vi "Initialize-intruments.vi"(0 "Initialize":bool, 1 "Status":T1={"CCD - Symphony Status 2"={"CCD - Status"="", "Error"=FALSE, "Initialized"=FALSE}, "Common: CCD 2"={"ID: CCD"=refnum, "Name"="ccd de test", "FirmwareVersion"="V1.89  CCD_3000", "activeXPixels"=1024, "activeYPixels"=256, "ADC Number"=[0], "ADC description"=[""], "Gain Number"=[0], "Gain description"=[""]}, "Monochromator - HR460 Status 2"={"Spectral Position"=0.0, "Spectral Unit"="", "Groove Density"=0.0, "Slit Width"=0.0, "Slit Unit"="", "Error"=FALSE, "Initialized"=FALSE}, "Stage - PI C844 Status 2"={" Identification Message "="", "Error"=FALSE, "Initialized"=FALSE}, "Temperature Controller - Status 2"={"Initialized"=FALSE, "Sample Temperature"=0.0, "Heater"=0, "Set Point"=20.0, "Error"=FALSE, "Sample Channel"=0, "Sample Channel Units"=0, "Unit"="Kelvin"}} {"Temperature Controller - Status 2"."Sample Channel Units" items=["Kelvin", "Celsius", "Sensor Units"]; "Temperature Controller - Status 2"."Sample Channel" items=["Sensor A", "Sensor B"]; "Temperature Controller - Status 2"."Heater" scale=0.0..100.0}, 5 "Instruments":T4, 7 "Monochromator - HR460 Control":T3, 9 "Stage - PI C844 Control":T6={" RS-232 Port Select "=0, " Interface Select "=1, "  P-term         I-term         D-term         Accel."=[[275, 120, 100, 2000000], [250, 40, 800, 2000000]]} {"Interface Select" items=["IEEE488", "RS-232"]; "RS-232 Port Select" items=["COM1", "COM2", "COM3", "COM4"]}, 11 "Temperature Controller - Control":T5={"VISA Resource Name"="GPIB0::12::INSTR", "Control Channel"=0, "Sample Channel Units"=0} {"Sample Channel Units" items=["Kelvin", "Celsius", "Sensor Units"]; "Control Channel" items=["Sensor A", "Sensor B"]}, 12 "error in (no error)":errorcluster) -> (3 "Common: CCD":T10={"ID: CCD"=refnum, "Name"="ccd de test", "FirmwareVersion"="V1.89  CCD_3000", "activeXPixels"=1024, "activeYPixels"=256, "ADC Number"=[], "ADC description"=[], "Gain Number"=[], "Gain description"=[]}, 4 "CCD - Symphony Status":T2, 6 "Shutter?":bool, 8 "Monochromator - HR460 Status":T9, 10 "Stage - PI C844 Status":T8, 14 "error out":errorcluster, 15 "Temperature Controller - Status":T7={"Initialized"=FALSE, "Sample Temperature"=0.0, "Heater"=0, "Set Point"=20.0, "Error"=FALSE, "Sample Channel"=0, "Sample Channel Units"=0, "Unit"="Kelvin"} {"Sample Channel Units" items=["Kelvin", "Celsius", "Sensor Units"]; "Sample Channel" items=["Sensor A", "Sensor B"]; "Heater" scale=0.0..100.0})   [LabVIEW 2009]
uses:
  lvmonos_LV7.1_all GPIB and RS232/Isa_user.llb/Spectrometer Status.GBL
  lvmonos_LV7.1_all GPIB and RS232/Isa_user.llb/SPECTROMETER SETUP.GBL
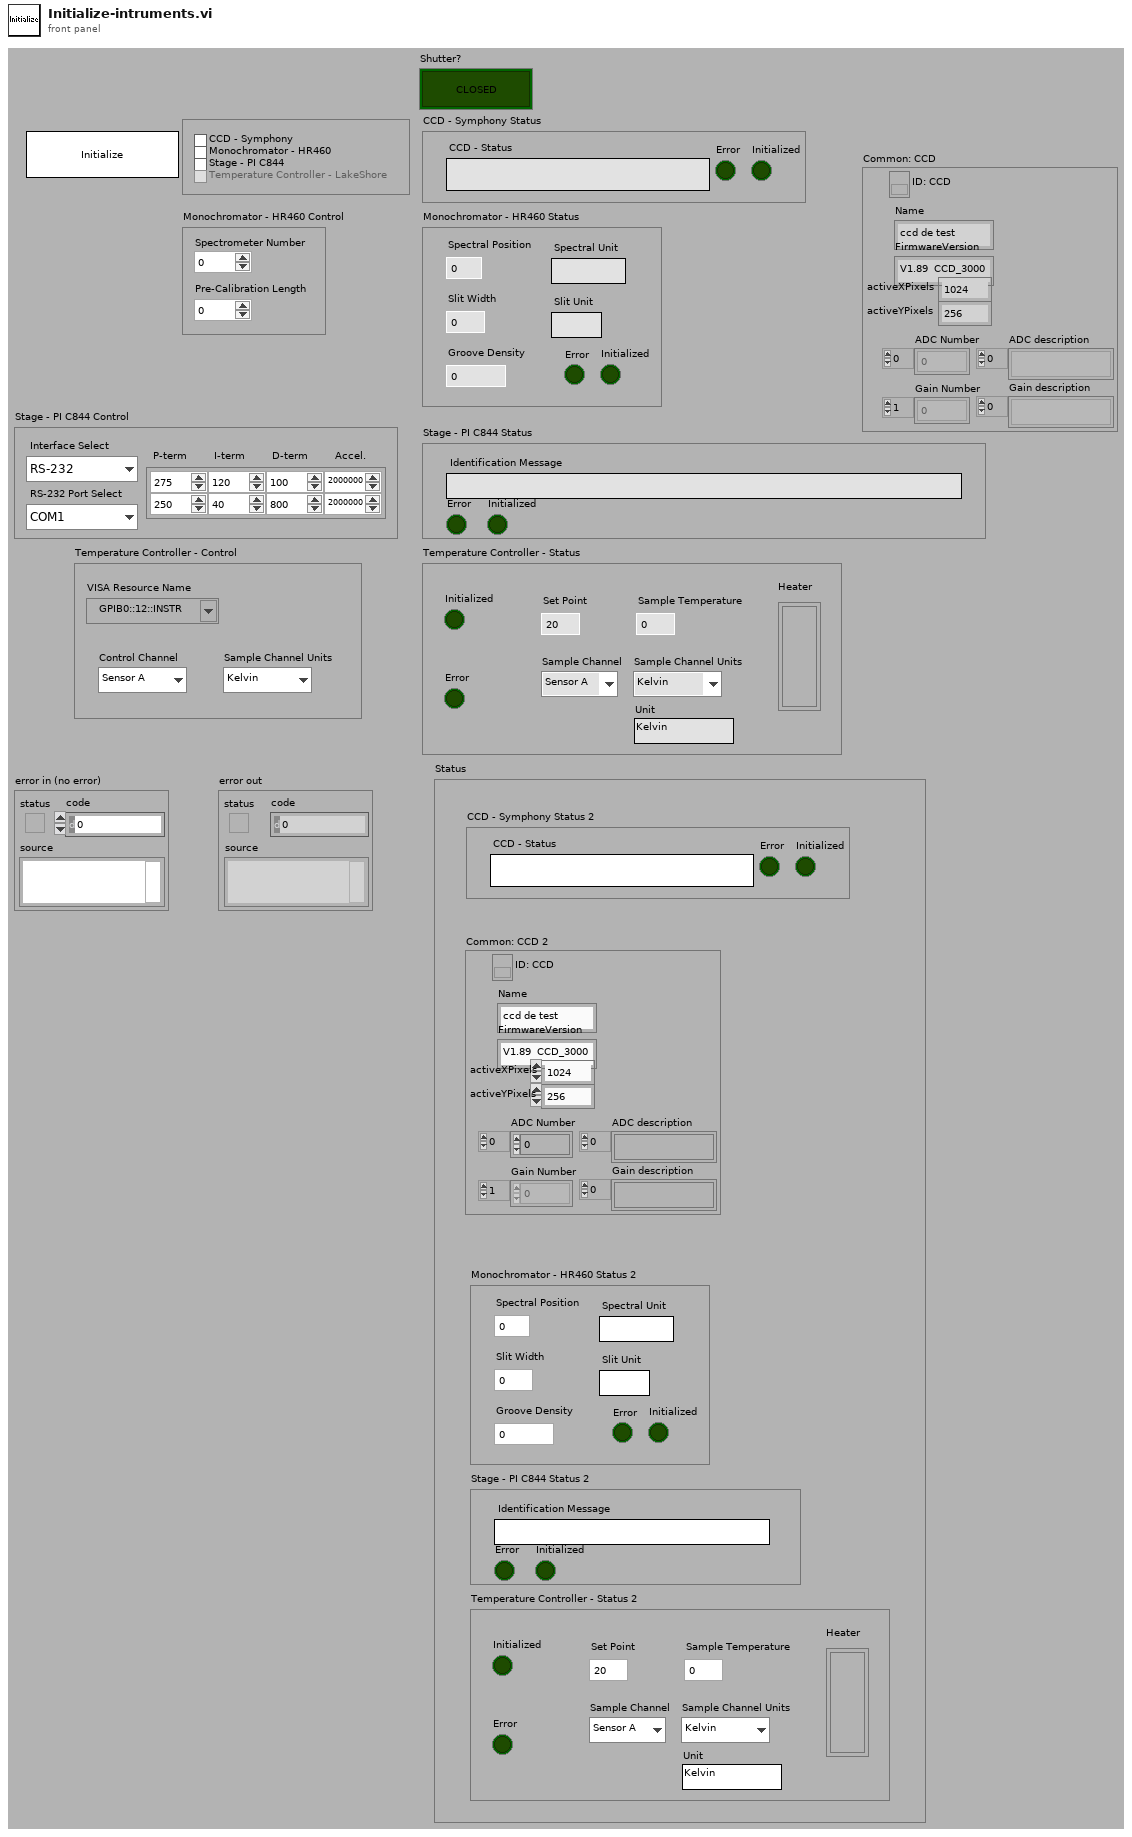
[diagram p1: front panel]
types:
  T1 = cluster{"CCD - Symphony Status 2":cluster{"CCD - Status":string, "Error":bool, "Initialized":bool}, "Common: CCD 2":cluster{"ID: CCD":refnum<k7>, "Name":string, "FirmwareVersion":string, "activeXPixels":i32, "activeYPixels":i32, "ADC Number":i32[], "ADC description":string[], "Gain Number":i32[], "Gain description":string[]}, "Monochromator - HR460 Status 2":cluster{"Spectral Position":dbl, "Spectral Unit":string, "Groove Density":dbl, "Slit Width":dbl, "Slit Unit":string, "Error":bool, "Initialized":bool}, "Stage - PI C844 Status 2":cluster{" Identification Message ":string, "Error":bool, "Initialized":bool}, "Temperature Controller - Status 2":cluster{"Initialized":bool, "Sample Temperature":dbl, "Heater":u8, "Set Point":dbl, "Error":bool, "Sample Channel":u16, "Sample Channel Units":u16, "Unit":string}}
  T2 = cluster{"CCD - Status":string, "Error":bool, "Initialized":bool}
  T3 = cluster{"Spectrometer Number":i32, "Pre-Calibration Length":dbl}
  T4 = cluster{"CCD - Symphony":bool, "Monochromator - HR460":bool, "Stage - PI C844":bool, "Temperature Controller - LakeShore":bool}
  T5 = cluster{"VISA Resource Name":refnum<visa-resource-name>, "Control Channel":u16, "Sample Channel Units":u16}
  T6 = cluster{" RS-232 Port Select ":i32, " Interface Select ":u8, "  P-term         I-term         D-term         Accel.":u32[][]}
  T7 = cluster{"Initialized":bool, "Sample Temperature":dbl, "Heater":u8, "Set Point":dbl, "Error":bool, "Sample Channel":u16, "Sample Channel Units":u16, "Unit":string}
  T8 = cluster{" Identification Message ":string, "Error":bool, "Initialized":bool}
  T9 = cluster{"Spectral Position":dbl, "Spectral Unit":string, "Groove Density":dbl, "Slit Width":dbl, "Slit Unit":string, "Error":bool, "Initialized":bool}
  T10 = cluster{"ID: CCD":refnum<k7>, "Name":string, "FirmwareVersion":string, "activeXPixels":i32, "activeYPixels":i32, "ADC Number":i32[], "ADC description":string[], "Gain Number":i32[], "Gain description":string[]}
  T11 = cluster{"Spectrometer Number":enum32{"Index Zero", "Index One"}, "Communication Parameters":cluster{"Comm Interface":u16, "GPIB Bus":i16, "GPIB Address":i16, "Serial Com Port":i32}, "Calibration":bool, "Groove Density":dbl[], "Blaze Wavelength":dbl[], "Base Grating":dbl, "Steps / Spectral Unit":dbl, "Backlash (Spectral Unit)":dbl, "Min Limit (Spectral Unit)":dbl, "Max Limit (Spectral Unit)":dbl, "Spectral Unit":string, "Slit Installation":cluster{"Axial Entrance":bool, "Lateral Entrance":bool, "Axial Exit":bool, "Lateral Exit":bool}, " Steps / Slit Unit":dbl, "Backlash (Slit Unit)":dbl, "Slit  Unit":string, " Max Limit (Slit Unit)":dbl, " Min Limit (Slit Unit)":dbl, "Drive Type":enum32{"Step", "Wavelength "}}[]
  T12 = cluster{"Spectrometer Number":enum32{"Index Zero", "Index One"}, "Communication Parameters":cluster{"Comm Interface":u16, "GPIB Bus":i16, "GPIB Address":i16, "Serial Com Port":i32}, "Calibration":bool, "Groove Density":dbl[], "Blaze Wavelength":dbl[], "Base Grating":dbl, "Steps / Spectral Unit":dbl, "Backlash (Spectral Unit)":dbl, "Min Limit (Spectral Unit)":dbl, "Max Limit (Spectral Unit)":dbl, "Spectral Unit":string, "Slit Installation":cluster{"Axial Entrance":bool, "Lateral Entrance":bool, "Axial Exit":bool, "Lateral Exit":bool}, " Steps / Slit Unit":dbl, "Backlash (Slit Unit)":dbl, "Slit  Unit":string, " Max Limit (Slit Unit)":dbl, " Min Limit (Slit Unit)":dbl, "Drive Type":enum32{"Step", "Wavelength "}}
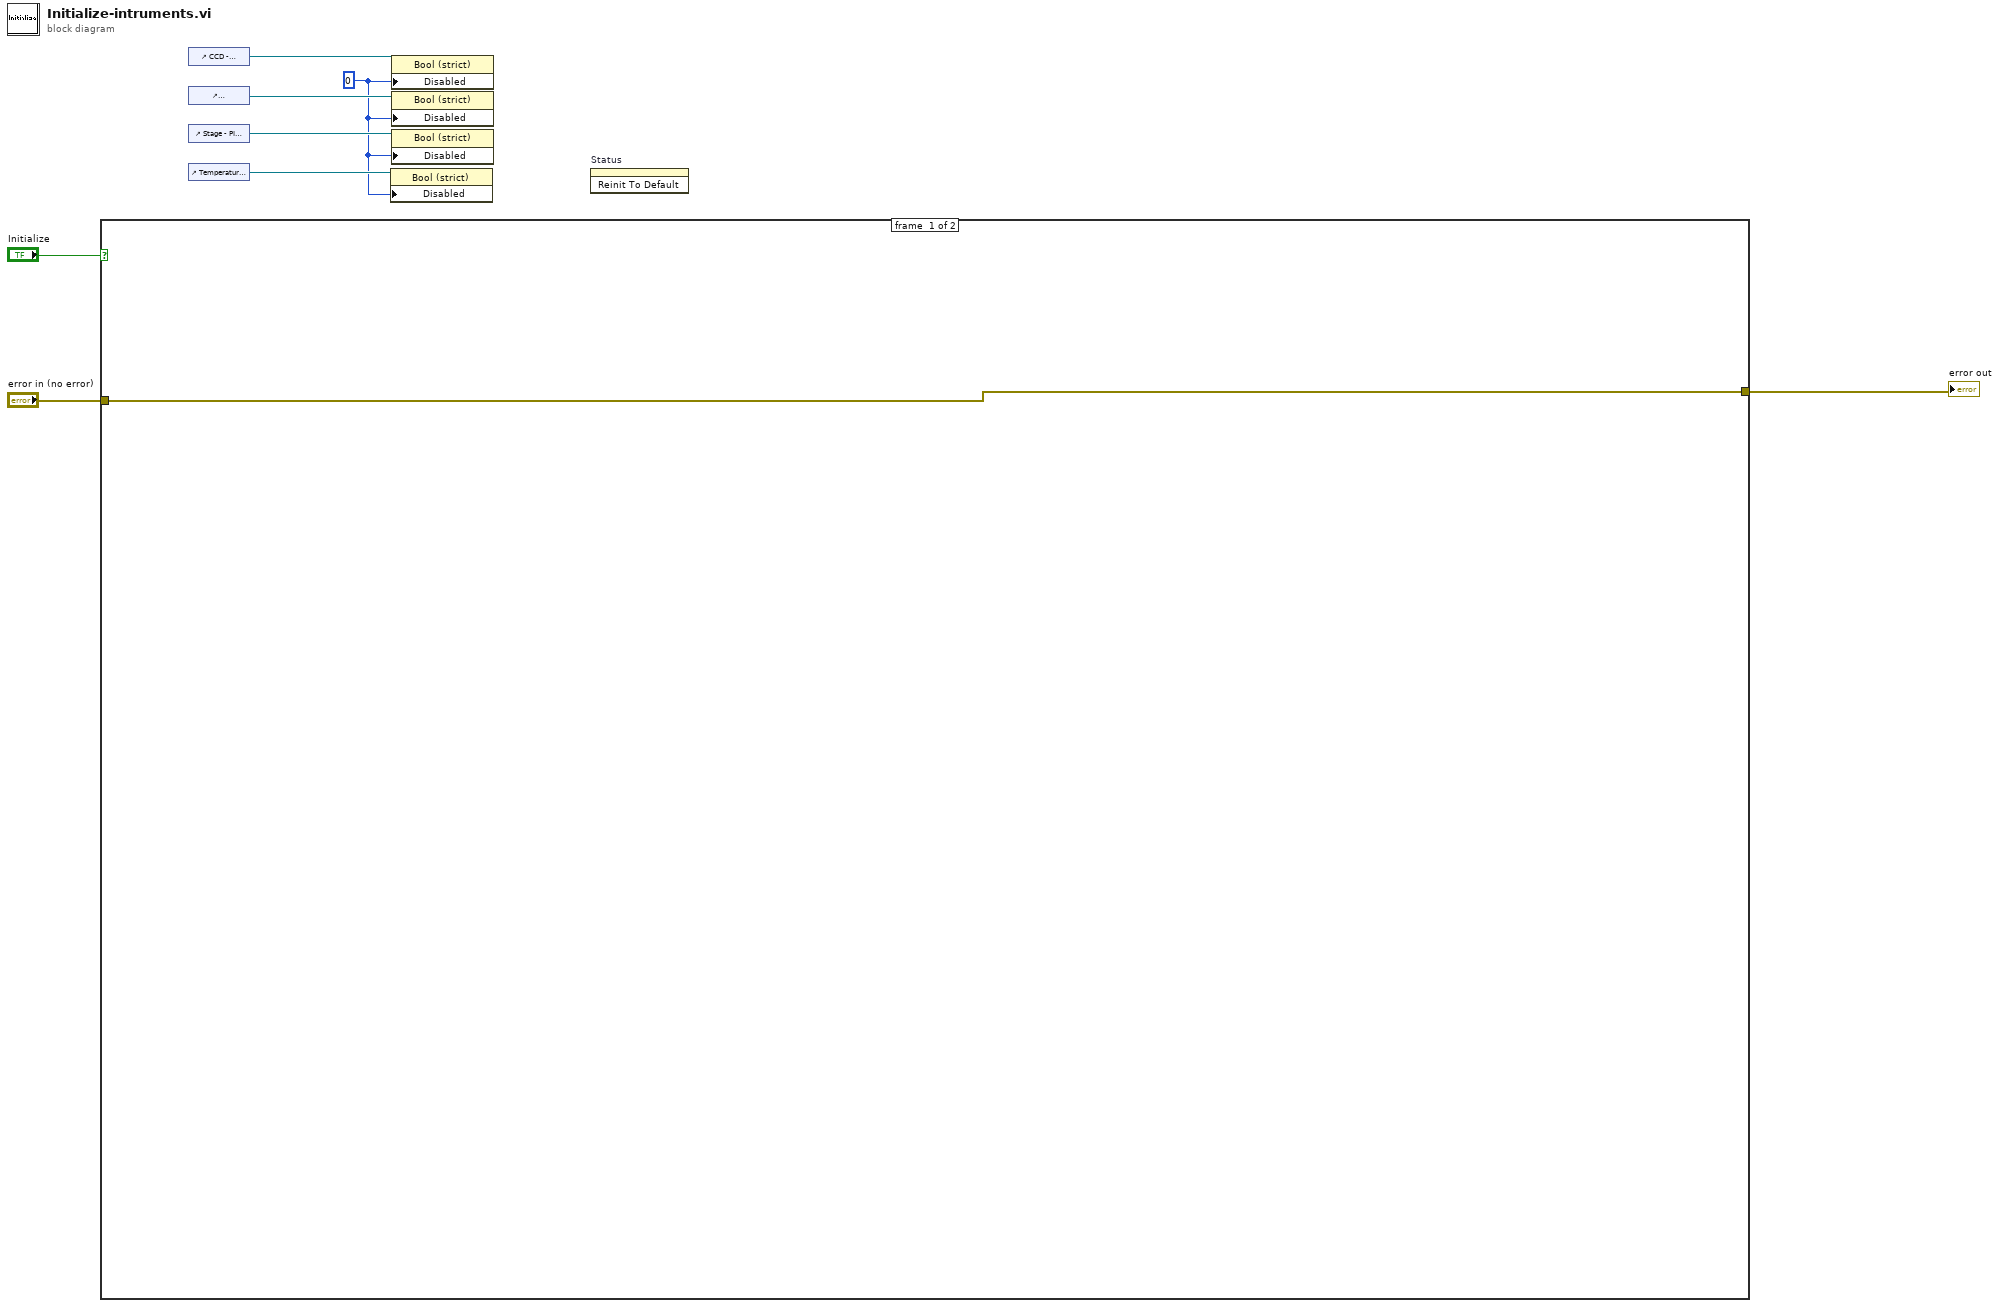
[diagram p0: block diagram]
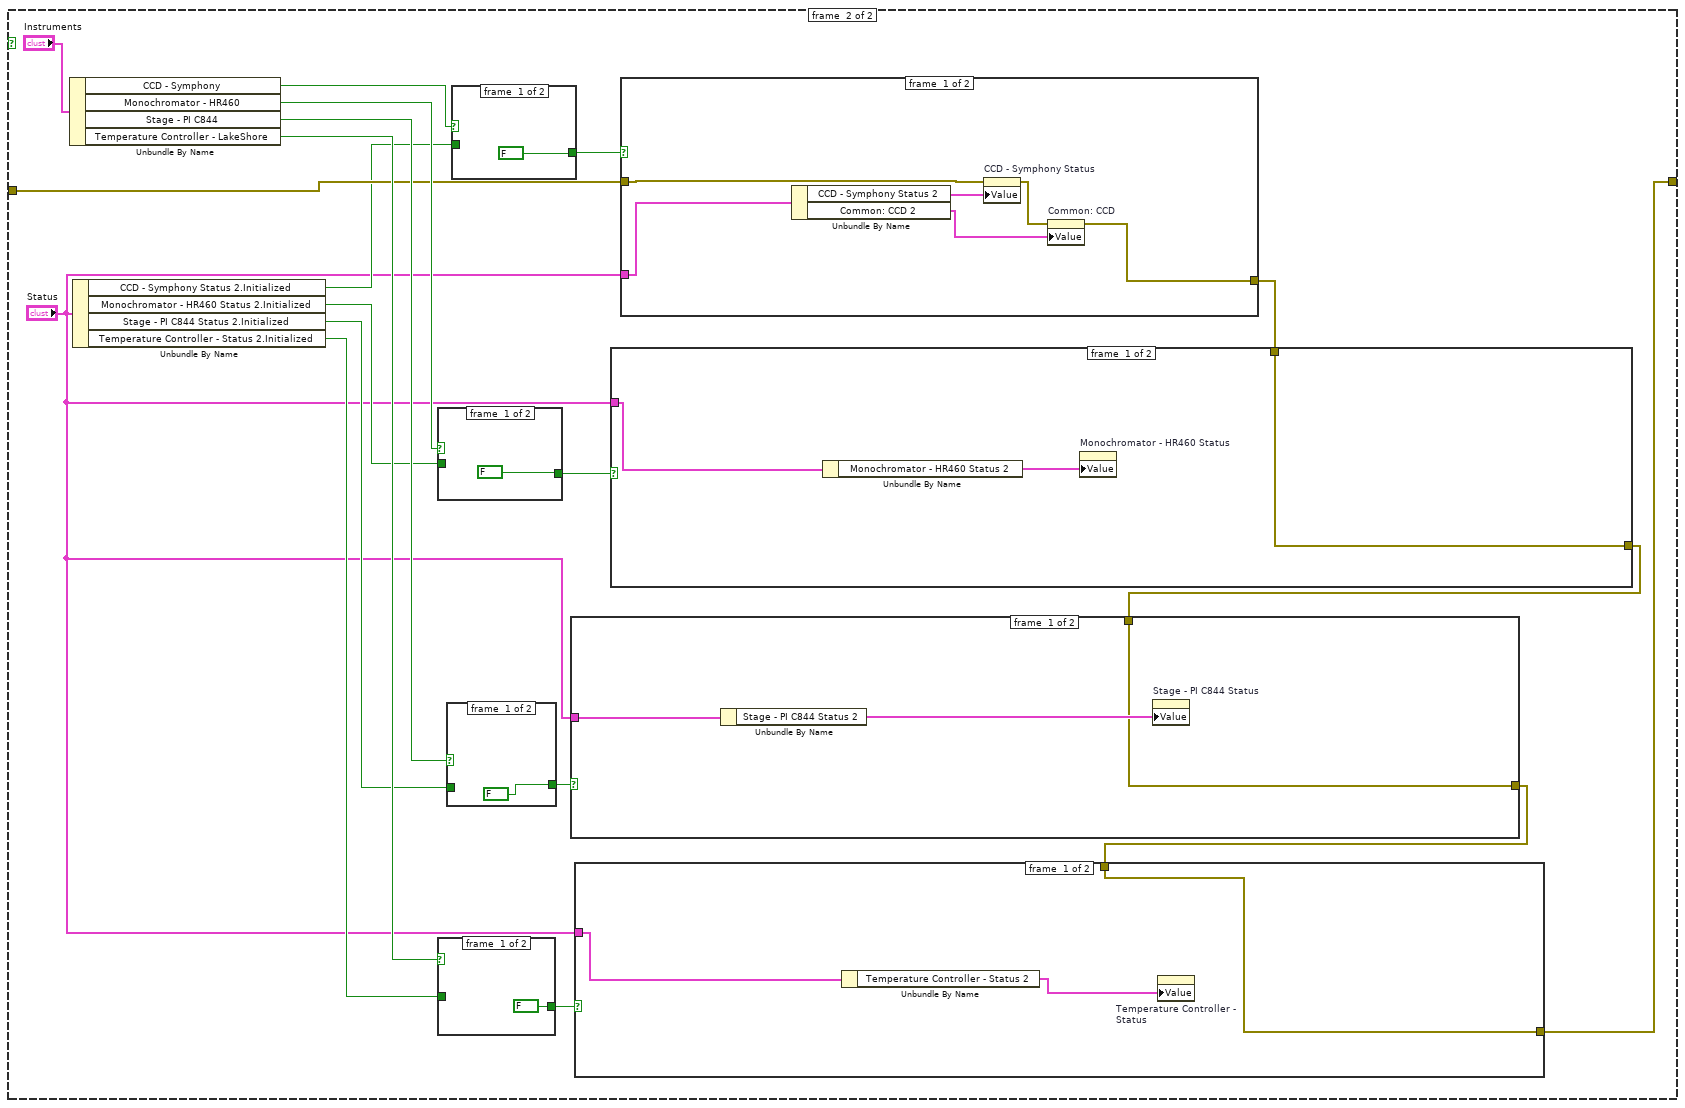
[diagram p2: hidden frame]
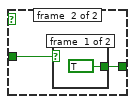
[diagram p3: hidden frame]
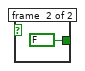
[diagram p4: hidden frame]
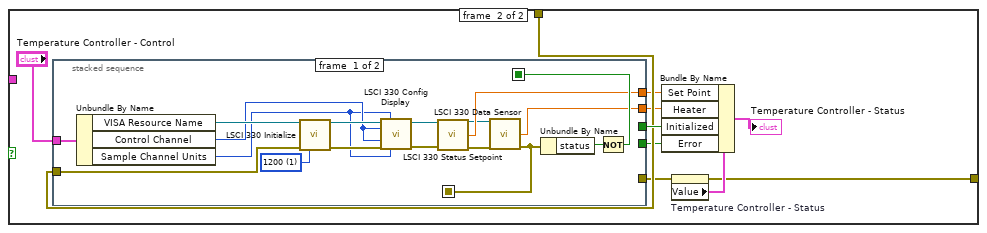
[diagram p5: hidden frame]
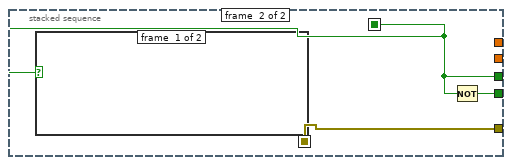
[diagram p6: hidden frame]
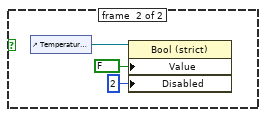
[diagram p7: hidden frame]
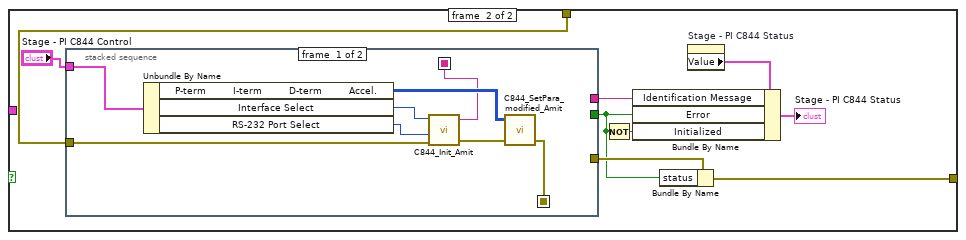
[diagram p8: hidden frame]
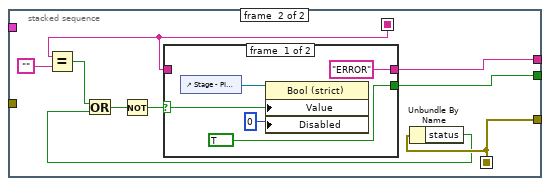
[diagram p9: hidden frame]
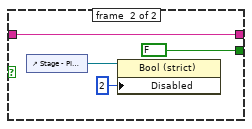
[diagram p10: hidden frame]
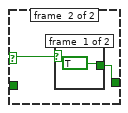
[diagram p11: hidden frame]
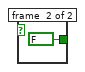
[diagram p12: hidden frame]
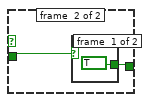
[diagram p13: hidden frame]
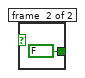
[diagram p14: hidden frame]
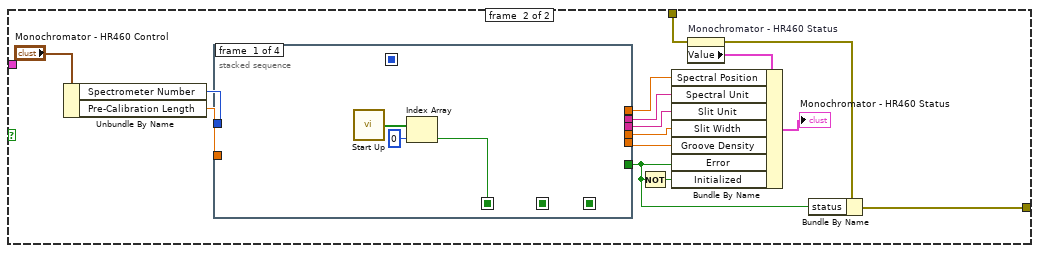
[diagram p15: hidden frame]
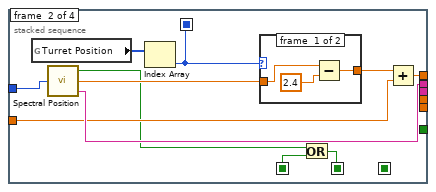
[diagram p16: hidden frame]
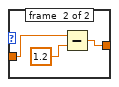
[diagram p17: hidden frame]
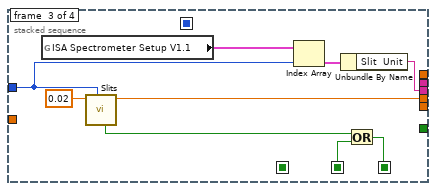
[diagram p18: hidden frame]
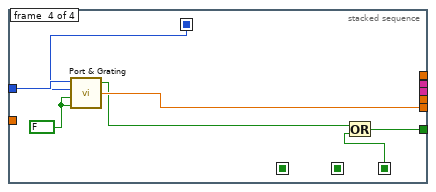
[diagram p19: hidden frame]
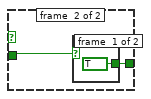
[diagram p20: hidden frame]
diagram:
  w1 = u8 0 ("Disabled")
  n1 = case shown="True" "Initialize" {
    tunnel: [w9 w15] -> w6
    tunnel: "error in (no error)" -> [w9 w23]
    frame #0 {
    }
    frame #1 {
      n2 = Unbundle By Name("Instruments") -> ("CCD - Symphony"=w24:bool, "Monochromator - HR460"=w25:bool, "Stage - PI C844"=w26:bool, "Temperature Controller - LakeShore"=w27:bool)
      n3 = Unbundle By Name("Status") -> ("CCD - Symphony Status 2.Initialized"=w14:bool, "Monochromator - HR460 Status 2.Initialized"=w13:bool, "Stage - PI C844 Status 2.Initialized"=w12:bool, "Temperature Controller - Status 2.Initialized"=w11:bool)
      n4 = case shown="False" w25 {
        tunnel: [FALSE w115] -> w21
        tunnel: w13 -> [_ w114]
        frame #0 {
        }
        frame #1 {
          n5 = case shown="True" w114 {
            tunnel: [TRUE FALSE] -> w115
            frame #0 {
            }
            frame #1 {
            }
          }
        }
      }
      n6 = case shown="False" w27 {
        tunnel: [FALSE w31] -> w19
        tunnel: w11 -> [_ w30]
        frame #0 {
        }
        frame #1 {
          n7 = case shown="True" w30 {
            tunnel: [TRUE FALSE] -> w31
            frame #0 {
            }
            frame #1 {
            }
          }
        }
      }
      n8 = case shown="True" w26 {
        tunnel: [FALSE w110] -> w20
        tunnel: w12 -> [_ w109]
        frame #0 {
        }
        frame #1 {
          n9 = case shown="False" w109 {
            tunnel: [TRUE FALSE] -> w110
            frame #0 {
            }
            frame #1 {
            }
          }
        }
      }
      n10 = case shown="False" w24 {
        tunnel: [FALSE w174] -> w22
        tunnel: w14 -> [_ w173]
        frame #0 {
        }
        frame #1 {
          n11 = case shown="False" w173 {
            tunnel: [TRUE FALSE] -> w174
            frame #0 {
            }
            frame #1 {
            }
          }
        }
      }
      n12 = case shown="True" w22 {
        tunnel: w23 -> [w180 w186]
        tunnel: [w177 w184] -> w18
        tunnel: "Status" -> [w182 _]
        frame #0 {
          n13 = Unbundle By Name(w182) -> ("CCD - Symphony Status 2"=w181:T2, "Common: CCD 2"=w179:T10)
          n14 = property on="CCD - Symphony Status" class="Clust (strict)"(error in=w180, "Value"=w181) -> (error out=w178:errorcluster)  [unwired: 1 in, 1 out]
          n15 = property on="Common: CCD" class="Clust (strict)"(error in=w178, "Value"=w179) -> (error out=w177:errorcluster)  [unwired: 1 in, 1 out]
        }
        frame #1 {
          n16 = stacked-sequence {
            seq-local: [_ w194 _] -> [_ _ w196]
            seq-local: [w187 _ _] -> [_ w191 _]
            tunnel: [_ _ w196] -> w185
            tunnel: w186 -> [w187 _ _]
            tunnel: [_ _ w195] -> w183
            frame #0 {
              w188 = FALSE
              n17 = Bundle("Initializing...", w188, w188) -> (→"CCD - Symphony Status":cluster{string, bool, bool})  [unwired: 1 in]
            }
            frame #1 {
              n18 = call "CCD Initialize-Amit.vi"("error in (no error)"=w191) -> ("error out"=w194:errorcluster, "Shutter?"=→"Shutter?":bool, "Common: CCD"=→"Common: CCD":T10)  [unwired: 7 in, 1 out]
            }
            frame #2 {
              n19 = Unbundle By Name(w196) -> ("status"=w195:bool)
              n20 = case shown="True" w195 {
                tunnel: w195 -> [w198 w204]
                frame #0 {
                  w197 = TRUE ("Value")
                  n21 = control-ref of="CCD - Symphony"() -> (w200:refnum<vi>)
                  n22 = property class="Bool (strict)"(reference=w200, "Disabled"=u8 2, "Value"=w197) -> ()  [unwired: 1 in, 2 out]
                  n23 = Bundle("CCD Initialized!!!  :-)", "status"=w198, "Value"=w197) -> (w202:cluster{string, "status":bool, "Value":bool})  [unwired: 1 in]
                  n24 = property on="CCD - Symphony Status" class="Clust (strict)"("Value"=w202) -> ()  [unwired: 2 in, 2 out]
                }
                frame #1 {
                  w203 = FALSE ("Value")
                  n25 = control-ref of="CCD - Symphony"() -> (w206:refnum<vi>)
                  n26 = property class="Bool (strict)"(reference=w206, "Value"=w203, "Disabled"=u8 0) -> ()  [unwired: 1 in, 2 out]
                  n27 = Bundle("Initialization Failed :-( ", "status"=w204, "Value"=w203) -> (w208:cluster{string, "status":bool, "Value":bool})  [unwired: 1 in]
                  n28 = property on="CCD - Symphony Status" class="Clust (strict)"("Value"=w208) -> ()  [unwired: 2 in, 2 out]
                }
              }
            }
          }
          n29 = Bundle By Name(cluster=w185, "status"=w183) -> (w184:errorcluster)
        }
      }
      n30 = case shown="False" w21 {
        tunnel: [w118 w121] -> w17
        tunnel: w18 -> [w118 w125]
        tunnel: "Status" -> [w120 _]
        frame #0 {
          n31 = Unbundle By Name(w120) -> ("Monochromator - HR460 Status 2"=w119:T9)
          n32 = property on="Monochromator - HR460 Status" class="Clust (strict)"("Value"=w119) -> ()  [unwired: 2 in, 2 out]
        }
        frame #1 {
          n33 = Unbundle By Name("Monochromator - HR460 Control") -> ("Spectrometer Number"=w127:i32, "Pre-Calibration Length"=w126:dbl)
          n34 = stacked-sequence {
            seq-local: [_ w146 _ _] -> [_ _ _ w170]
            seq-local: [w136 _ _ _] -> [_ w141 _ _]
            seq-local: [_ w139 _ _] -> [_ _ w158 _]
            seq-local: [_ _ w156 _] -> [_ _ _ w166]
            tunnel: w127 -> [_ w147 w162 w171]
            tunnel: [_ w144 _ _] -> w135
            tunnel: [_ w143 _ _] -> w134
            tunnel: [_ _ w160 _] -> w133
            tunnel: [_ _ w159 _] -> w132
            tunnel: [_ _ _ w168] -> w131
            tunnel: w126 -> [_ w142 _ _]
            tunnel: [_ _ _ w165] -> w122
            frame #0 {
              n35 = call "Start Up.VI"() -> ("Error List"=w138:bool[])  [unwired: 1 in, 2 out]
              n36 = Index Array(array=w138, index=0) -> (element=w136:bool)
            }
            frame #1 {
              n37 = global read "Spectrometer Status.GBL" "Turret Position"() -> (w149:i32[])
              n38 = call "Spectral Position.VI"("Spectrometer Number"=w147) -> ("Error"=w140:bool, "Present Position"=w148:dbl, "Spectral Unit"=w143:string)
              n39 = Index Array(array=w149) -> (element=w146:i32)  [unwired: 1 in]
              n40 = case shown="1, Default" w146 {
                tunnel: [w152 w154] -> w145
                tunnel: w148 -> [w151 w153]
                frame #0 {
                  n41 = Subtract(x=w151, y=2.4) -> (x-y=w152:dbl)
                }
                frame #1 {
                  n42 = Subtract(x=w153, y=1.2) -> (x-y=w154:dbl)
                }
              }
              n43 = Or(x=w140, y=w141) -> (x .or. y?=w139:bool)
              n44 = Add(x=w145, y=w142) -> (x+y=w144:dbl)
            }
            frame #2 {
              n45 = global read "SPECTROMETER SETUP.GBL" "ISA Spectrometer Setup V1.1"() -> (w163:T11)
              n46 = call "Slits.VI"("Spectrometer Number"=w162, "Axial Entrance"=0.02) -> ("Axial Entrance"=w159:dbl, "Error"=w157:bool)  [unwired: 3 in, 3 out]
              n47 = Index Array(array=w163, index=w162) -> (element=w161:T12)
              n48 = Unbundle By Name(w161) -> ("Slit  Unit"=w160:string)
              n49 = Or(x=w157, y=w158) -> (x .or. y?=w156:bool)
            }
            frame #3 {
              w169 = FALSE
              n50 = call "Port & Grating.VI"("Exit Mirror Pos"=w169, "Entrance Mirror Pos"=w169, "Turret Pos"=w170, "Spectrometer Number"=w171) -> ("Groove Density"=w168:dbl, "Error"=w167:bool)  [unwired: 1 out]
              n51 = Or(x=w167, y=w166) -> (x .or. y?=w165:bool)
            }
          }
          n52 = Not(x=w122) -> (.not. x?=w124:bool)
          n53 = property on="Monochromator - HR460 Status" class="Clust (strict)"(error in=w125) -> (error out=w123:errorcluster, "Value"=w129:T9)  [unwired: 1 in, 1 out]
          n54 = Bundle By Name(cluster=w129, "Spectral Position"=w135, "Spectral Unit"=w134, "Slit Unit"=w133, "Slit Width"=w132, "Groove Density"=w131, "Error"=w122, "Initialized"=w124) -> (→"Monochromator - HR460 Status":T9)
          n55 = Bundle By Name(cluster=w123, "status"=w122) -> (w121:errorcluster)
        }
      }
      n56 = case shown="True" w20 {
        tunnel: w17 -> [w70 w80]
        tunnel: [w70 w73] -> w16
        tunnel: "Status" -> [w72 _]
        frame #0 {
          n57 = Unbundle By Name(w72) -> ("Stage - PI C844 Status 2"=w71:T8)
          n58 = property on="Stage - PI C844 Status" class="Clust (strict)"("Value"=w71) -> ()  [unwired: 2 in, 2 out]
        }
        frame #1 {
          n59 = stacked-sequence {
            seq-local: [w83 _] -> [_ w90]
            seq-local: [w85 _] -> [_ w98]
            tunnel: "Stage - PI C844 Control" -> [w89 _]
            tunnel: [_ w96] -> w81
            tunnel: w80 -> [w86 _]
            tunnel: [_ w98] -> w75
            tunnel: [_ w95] -> w74
            frame #0 {
              n60 = Unbundle By Name(w89) -> ("P-term         I-term         D-term         Accel."=w84:u32[][], "Interface Select"=w88:u8, "RS-232 Port Select"=w87:i32)
              n61 = call "C844_Init_Amit.vi"("Error in"=w86, "RS-232 Port Select"=w87, "Interface Select"=w88) -> ("Error out"=w82:errorcluster, "Identification Message"=w83:string)  [unwired: 2 in]
              n62 = call "C844_SetPara_modified_Amit.vi"("Error in"=w82, "P-term   i-term   d-term   Accel."=w84) -> ("Error out"=w85:errorcluster)  [unwired: 3 in]
            }
            frame #1 {
              n63 = Equal?(x=w90, y="") -> (x = y?=w93:bool)
              n64 = Unbundle By Name(w98) -> ("status"=w92:bool)
              n65 = Or(x=w93, y=w92) -> (x .or. y?=w91:bool)
              n66 = Not(x=w91) -> (.not. x?=w97:bool)
              n67 = case shown="False" w97 {
                selector: w97 -> [w100 _]
                tunnel: w90 -> [_ w105]
                tunnel: ["ERROR" w105] -> w96
                tunnel: [TRUE FALSE] -> w95
                frame #0 {
                  n68 = control-ref of="Stage - PI C844"() -> (w103:refnum<vi>)
                  n69 = property class="Bool (strict)"(reference=w103, "Value"=w100, "Disabled"=u8 0) -> ()  [unwired: 1 in, 2 out]
                }
                frame #1 {
                  n70 = control-ref of="Stage - PI C844"() -> (w107:refnum<vi>)
                  n71 = property class="Bool (strict)"(reference=w107, "Disabled"=u8 2) -> ()  [unwired: 1 in, 2 out]
                }
              }
            }
          }
          n72 = Not(x=w74) -> (.not. x?=w76:bool)
          n73 = Bundle By Name(cluster=w75, "status"=w74) -> (w73:errorcluster)
          n74 = property on="Stage - PI C844 Status" class="Clust (strict)"() -> ("Value"=w77:T8)  [unwired: 2 in, 2 out]
          n75 = Bundle By Name(cluster=w77, "Identification Message"=w81, "Error"=w74, "Initialized"=w76) -> (→"Stage - PI C844 Status":T8)
        }
      }
      n76 = case shown="True" w19 {
        tunnel: w16 -> [w34 w45]
        tunnel: [w34 w40] -> w15
        tunnel: "Status" -> [w36 _]
        frame #0 {
          n77 = Unbundle By Name(w36) -> ("Temperature Controller - Status 2"=w35:T7)
          n78 = property on="Temperature Controller - Status" class="Clust (strict)"("Value"=w35) -> ()  [unwired: 2 in, 2 out]
        }
        frame #1 {
          n79 = stacked-sequence {
            seq-local: [w54 _] -> [_ w65]
            seq-local: [w53 _] -> [_ w66]
            tunnel: [_ w65] -> w46
            tunnel: w45 -> [w56 _]
            tunnel: [_ w66] -> w41
            tunnel: "Temperature Controller - Control" -> [w55 _]
            tunnel: [_ w64] -> w39
            tunnel: [w47 _] -> w38
            tunnel: [w50 _] -> w37
            frame #0 {
              w61 = 1 items=["300", "1200"] ("Baud Rate [1: 1200]")
              n80 = Unbundle By Name(w55) -> ("VISA Resource Name"=w63:refnum<visa-resource-name>, "Control Channel"=w59:u16, "Sample Channel Units"=w57:u16)
              n81 = call "LSCI 330 Initialize.vi"("VISA Resource Name"=w63, "error in (no error)"=w56, "Baud Rate [1: 1200]"=w61) -> ("VISA session"=w62:refnum<visa-resource-name>, "error out"=w60:errorcluster)  [unwired: 11 in]
              n82 = call "LSCI 330 Config Display.vi"("VISA session"=w62, "Control Channel Units (0: Kelvin)"=w57, "Control Channel (0: Sensor A)"=w59, "Sample Channel (0: Sensor A)"=w59, "error in (no error)"=w60, "Sample Channel Units (0: Kelvin)"=w57) -> ("dup VISA session"=w48:refnum<visa-resource-name>, "error out"=w52:errorcluster)  [unwired: 8 in]
              n83 = call "LSCI 330 Status Setpoint.vi"("VISA session"=w48, "error in (no error)"=w52) -> ("dup VISA session"=w49:refnum<visa-resource-name>, "Setpoint"=w50:dbl, "error out"=w51:errorcluster)  [unwired: 11 in]
              n84 = call "LSCI 330 Data Sensor.vi"("VISA session"=w49, "error in (no error)"=w51) -> ("Control Sensor Data"=w47:dbl, "error out"=w53:errorcluster)  [unwired: 10 in, 2 out]
              n85 = Unbundle By Name(w53) -> ("status"=w58:bool)
              n86 = Not(x=w58) -> (.not. x?=w54:bool)
            }
            frame #1 {
              n87 = case shown="True" w65 {
                frame #0 {
                }
                frame #1 {
                  n88 = control-ref of="Temperature Controller - LakeShore"() -> (w67:refnum<vi>)
                  n89 = property class="Bool (strict)"(reference=w67, "Value"=FALSE, "Disabled"=u8 2) -> ()  [unwired: 1 in, 2 out]
                }
              }
              n90 = Not(x=w65) -> (.not. x?=w64:bool)
            }
          }
          n91 = property on="Temperature Controller - Status" class="Clust (strict)"(error in=w41) -> (error out=w40:errorcluster, "Value"=w43:T7)  [unwired: 1 in, 1 out]
          n92 = Bundle By Name(cluster=w43, "Set Point"=w37, "Heater"=w38, "Initialized"=w46, "Error"=w39) -> (→"Temperature Controller - Status":T7)
        }
      }
    }
  }
  "error out" <- w6
  n93 = control-ref of="CCD - Symphony"() -> (w5:refnum<vi>)
  n94 = control-ref of="Monochromator - HR460"() -> (w4:refnum<vi>)
  n95 = control-ref of="Stage - PI C844"() -> (w3:refnum<vi>)
  n96 = control-ref of="Temperature Controller - LakeShore"() -> (w2:refnum<vi>)
  n97 = property class="Bool (strict)"(reference=w2, "Disabled"=w1) -> ()  [unwired: 1 in, 2 out]
  n98 = property class="Bool (strict)"(reference=w5, "Disabled"=w1) -> ()  [unwired: 1 in, 2 out]
  n99 = property class="Bool (strict)"(reference=w4, "Disabled"=w1) -> ()  [unwired: 1 in, 2 out]
  n100 = property class="Bool (strict)"(reference=w3, "Disabled"=w1) -> ()  [unwired: 1 in, 2 out]
  n101 = invoke on="Status" class="Clust (strict)" method="Reinit To Default"() -> ()  [unwired: 3 in, 3 out]
